vi "image_avg_no_reshape.vi"(9 "Numeric":dbl, 10 "points / pixel":i32, 11 "input array":dbl[][](array[numeric])) -> (3 "output array":dbl[][](array[numeric]))   [LabVIEW 2014]
panel:
  out "average element":dbl
  out "dim 2":i32
  out "dim 1":i32
  out "dim 2":i32
  out "dim 1":i32
  # "Input"
  # "Output"
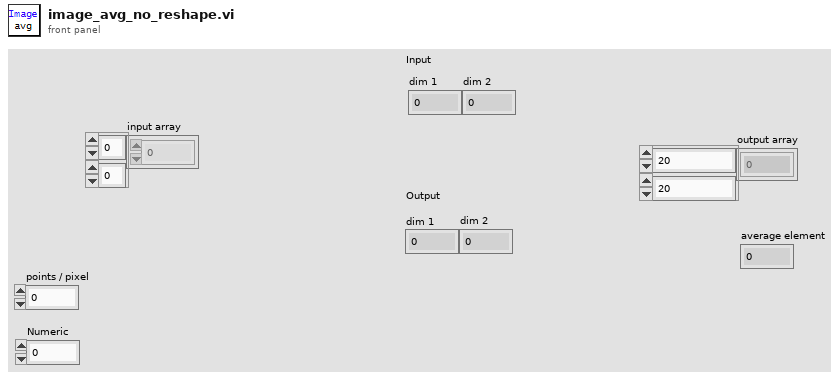
[diagram p1: front panel]
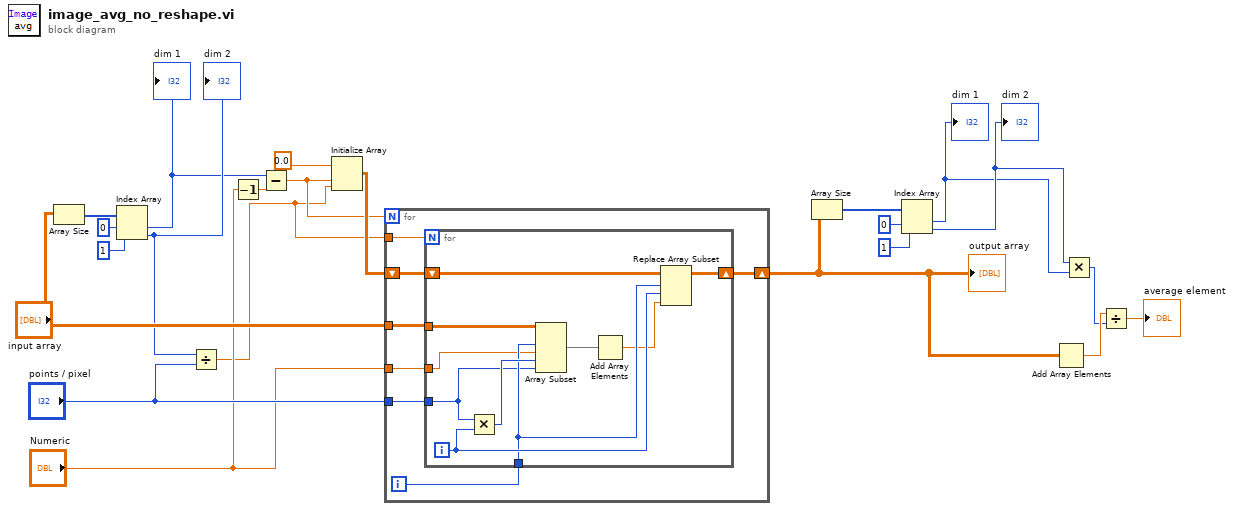
[diagram p0: block diagram]
diagram:
  n1 = Array Size(array="input array") -> (size(s)=w20:i32[])
  n2 = Index Array(array=w20, index #1=0 ("index"), index #2=1 ("index")) -> (element #1=w14:i32, element #2=w15:i32)
  "dim 1" <- w14
  "dim 2" <- w15
  n3 = Divide(x=w15, y="points / pixel") -> (x/y=w10:dbl)
  n4 = Decrement(x="Numeric") -> (x-1=w13:dbl)
  n5 = Subtract(x=w14, y=w13) -> (x-y=w11:dbl)
  n6 = Initialize Array(0.0 ("element"), w11, w10) -> (w21:dbl[][])
  n7 = for {
    N: w11 -> [_]
    shift-right: [w29] -> w6
    shift-left: w21 -> [w28]
    tunnel: "points / pixel" -> [w24]
    tunnel: "Numeric" -> [w26]
    tunnel: "input array" -> [w27]
    tunnel: w10 -> [w25]
    i -> [w23]
    n8 = for {
      N: w25 -> [_]
      tunnel: w27 -> [w37]
      tunnel: w26 -> [w31]
      shift-right: [w39] -> w29
      shift-left: w28 -> [w38]
      tunnel: w24 -> [w30]
      tunnel: w23 -> [w33]
      i -> [w34]
      n9 = Multiply(x=w30, y=w34) -> (x*y=w35:i32)
      n10 = Array Subset(array=w37, index (row)=w33, length (row)=w31, index (col)=w35, length (col)=w30) -> (w36:dbl[][])
      n11 = Add Array Elements(numeric array=w36) -> (sum=w32:dbl)
      n12 = Replace Array Subset(array=w38, new element=w32, index (row)=w33, index (col)=w34) -> (w39:dbl[][])
    }
  }
  "output array" <- w6
  n13 = Array Size(array=w6) -> (size(s)=w7:i32[])
  n14 = Index Array(array=w7, index #1=0 ("index"), index #2=1 ("index")) -> (element #1=w4:i32, element #2=w5:i32)
  "dim 1" <- w4
  "dim 2" <- w5
  n15 = Add Array Elements(numeric array=w6) -> (sum=w3:dbl)
  n16 = Multiply(x=w5, y=w4) -> (x*y=w2:i32)
  n17 = Divide(x=w3, y=w2) -> (x/y=→"average element":dbl)
